vi "connect_network.vi"(8 "error in":errorcluster, 9 "Network params":T1={"Remote Host"="192.168.1.3", "Send Status"=TRUE, "Send Port"=61557, "Recv Commands"=FALSE, "Recv Port"=0}) -> (0 "error out":errorcluster, 1 "Host Addr":u32, 2 "Recv UDP Conn":refnum<k16>, 3 "Send UDP Conn":refnum<k16>)   [LabVIEW 2014]
uses:
  network_params.ctl
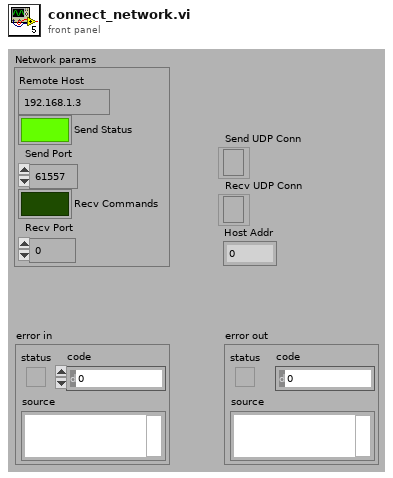
[diagram p1: front panel]
types:
  T1 = typedef "network_params.ctl" = cluster{"Remote Host":string, "Send Status":bool, "Send Port":u16, "Recv Commands":bool, "Recv Port":u16}
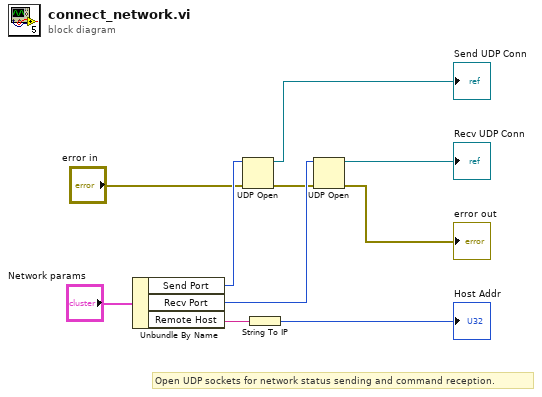
[diagram p0: block diagram]
diagram:
  # "Open UDP sockets for network status sending and command reception."
  n1 = Unbundle By Name("Network params") -> ("Send Port"=w7:u16, "Recv Port"=w8:u16, "Remote Host"=w10:string)
  n2 = UDP Open(8:"error in", 11:w7) -> (port=→"Send UDP Conn":refnum<k16>, 0:w2:errorcluster)  [unwired: 4 out]
  n3 = String To IP(1:w10) -> (0:→"Host Addr":u32)
  n4 = UDP Open(8:w2, 11:w8) -> (port=→"Recv UDP Conn":refnum<k16>, 0:→"error out":errorcluster)  [unwired: 4 out]
